vi "ReportError.vi"(8 "error in (no error)":errorcluster, 10 "ErrorReported":errorcluster, 11 "ModuleID":i32) -> (0 "error out":errorcluster)   [LabVIEW 2018, in "MyPlugins.lvlib"]
doc: "Broadcasts any error from the module."
uses:
  MyPlugins/MyPlugins.lvlib
  clEventType.ctl
  PluginsShared.lvlib
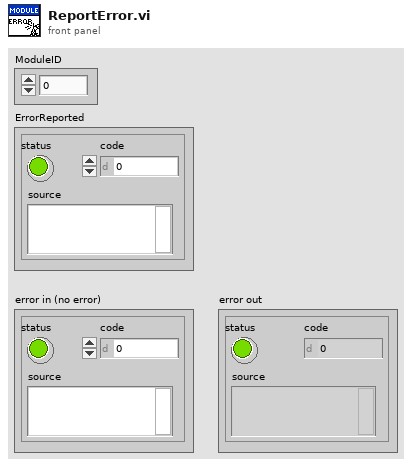
[diagram p1: front panel]
types:
  T1 = typedef "PluginsShared.lvlib/clEventType.ctl" = cluster{"ModuleID":i32, "Data":variant}
  T2 = typedef "PluginsShared.lvlib/clBroadcastEvents.ctl" = cluster{"DidInit":refnum<user-event>, "StatusUpdate":refnum<user-event>, "ErrorReport":refnum<user-event>, "DidStop":refnum<user-event>, "PathToINI":refnum<user-event>, "ReloadINIFiles":refnum<user-event>}
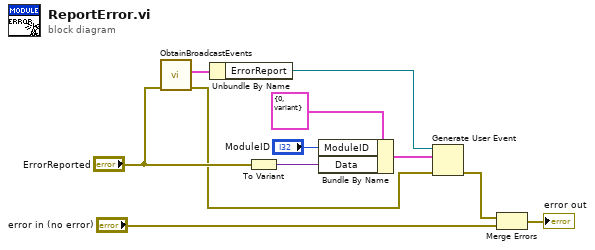
[diagram p0: block diagram]
diagram:
  n1 = call "ObtainBroadcastEvents.vi"("error in (no error)"="ErrorReported") -> ("error out"=w3:errorcluster, "clBroadcastEvents"=w8:T2)  [unwired: 9 in]
  n2 = Unbundle By Name(w8) -> ("ErrorReport"=w6:refnum<user-event>)
  n3 = To Variant(anything="ErrorReported") -> (Variant=w10:variant)
  n4 = Bundle By Name(cluster=T1 {"ModuleID"=0, "Data"=variant} ("clEventType"), "ModuleID"="ModuleID", "Data"=w10) -> (w7:T1)
  n5 = Generate User Event(user event=w6, event data cluster=w7, error in=w3) -> (error out=w1:errorcluster)  [unwired: 1 in, 1 out]
  n6 = Merge Errors(w1, "error in (no error)") -> (→"error out":errorcluster)
